vi "Material-ConfigDialog-Destroy.vi"(0 "Configuration Dialog":refnum<class "Material-ConfigDialog.lvclass">, 11 "error in":errorcluster) -> (15 "error out":errorcluster)   [LabVIEW 2013, in "Material-ConfigDialog.lvclass"]
uses:
  Material-ConfigDialog.lvclass
  Material-ConfigDialog.lvclass/Material-ConfigDialog.ctl
  Reuse Library/featherweight/Core/Messaging/Messenger.Actor/FTW-Messenger-Actor.lvclass
panel:
  # "Inputs"
  # "Outputs"
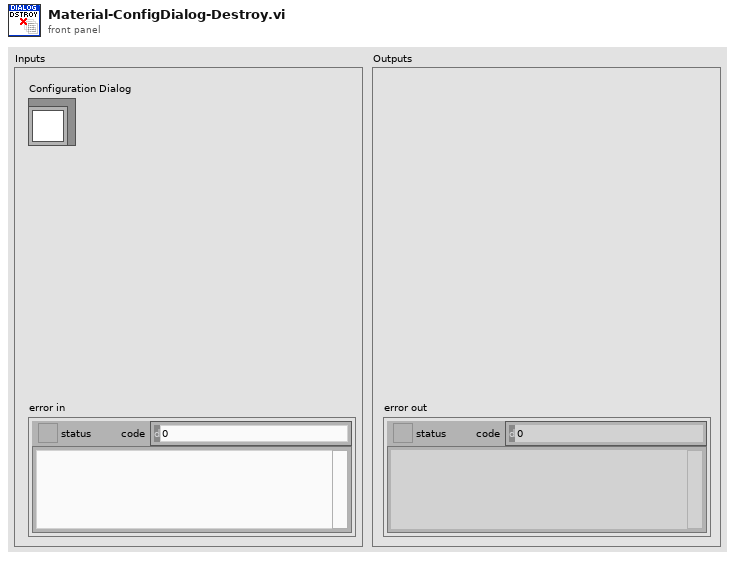
[diagram p1: front panel]
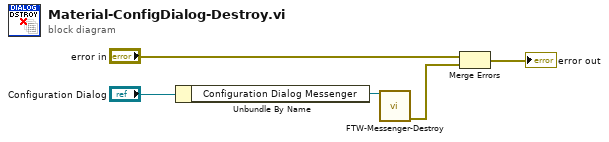
[diagram p0: block diagram]
diagram:
  n1 = Unbundle By Name("Configuration Dialog") -> ("Configuration Dialog Messenger"=w2:refnum<class "FTW-Messenger-Actor.lvclass">)
  n2 = call-dynamic "FTW-Messenger-Destroy.vi"("Messenger"=w2) -> ("error out"=w1:errorcluster)  [unwired: 14 in]
  n3 = Merge Errors("error in", w1) -> (→"error out":errorcluster)
